vi "Send Show_GUI.vi"(7 "Message Priority (Normal)":T1=enum."Normal" caption="Priorité des messages (normale)", 8 "error in (no error)":errorcluster caption="entrée d'erreur (pas d'erreur)", 10 "Show_GUI":bool=TRUE, 11 "Message Enqueuer":refnum<class "Message Enqueuer.lvclass"> caption="Objet ajoutant des msgs à la file") -> (0 "error out":errorcluster caption="sortie d'erreur", 3 "Message Enqueuer out":refnum<class "Message Enqueuer.lvclass"> caption="Objet ajoutant des msgs à la file en sortie")   [LabVIEW 2020, in "Library Core.lvlib" / "Actor_EventStart.lvlib" / "Message Show_GUI.lvclass"]
doc: "Ce VI envoie le message à un acteur."
uses:
  Message Show_GUI.lvclass
  <vilib>/ActorFramework/Message Enqueuer/Message Enqueuer.lvclass
  <vilib>/ActorFramework/Message Enqueuer/Message Priority.ctl
  C:/Program Files (x86)/National Instruments/LabVIEW 2020/vi.lib/ActorFramework/Message/Message.lvclass
  Message Show_GUI.lvclass/Message Show_GUI.ctl
  <vilib>/ActorFramework/Message Enqueuer/Message Enqueuer.lvclass/Message Enqueuer.ctl
  <vilib>/ActorFramework/Message Priority Queue/Priority Enqueue.vi
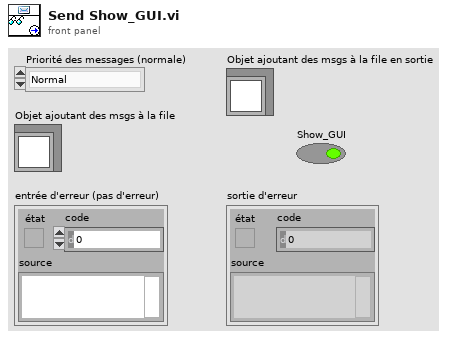
[diagram p1: front panel]
types:
  T1 = typedef "Actor Framework.lvlib/Message Enqueuer.lvclass/Message Priority.ctl" = enum16{"Low", "Normal", "High"}
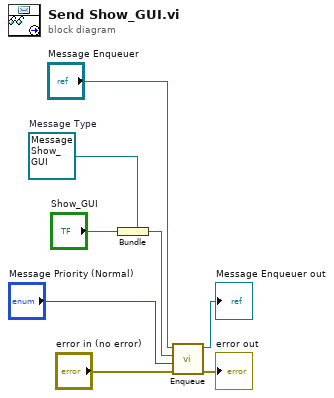
[diagram p0: block diagram]
diagram:
  w3 = refnum<class "Message Show_GUI.lvclass"> refnum  # Message Type
  n1 = Bundle(cluster=w3, "Show_GUI") -> (w1:refnum<class "Message Show_GUI.lvclass">)
  n2 = call <vilib>:"Enqueue.vi"("error in (no error)"="error in (no error)", "Message Priority (Normal)"="Message Priority (Normal)", "Message"=w1, "Message Enqueuer in"="Message Enqueuer") -> ("error out"=→"error out":errorcluster, "Message Enqueuer out"=→"Message Enqueuer out":refnum<class "Message Enqueuer.lvclass">)  [unwired: 6 in]
